vi "poly_time_conversion_ms2s_single.vi"(2 "ms":i32) -> (7 "s":dbl format="%#_13g")   [LabVIEW 2015]
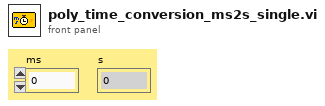
[diagram p1: front panel]
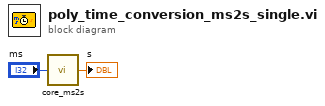
[diagram p0: block diagram]
diagram:
  n1 = call "core_ms2s.vi"("ms"="ms") -> ("s"=→"s":dbl)  [unwired: 8 in]
